vi "Test-DriveForwardDistance-DMR.vi"(9 "TestProgress NT":string, 10 "TestProgressText NT":string, 11 "TestName NT":string) -> ()   [LabVIEW 2013]
uses:
  Systems/DriveMotors/DriveMotors.lvclass
  Commands/DM-DriveForwardDistance/DM-DriveForwardDistance.lvclass
  Commands/Command/Command.lvclass
  Robot Global Data.vi
panel:
  in  "Test Wait":u32=25
  in  "DrivePower":dbl=0.4 format="%#_13g"
  in  "DistanceToDrive":dbl=600.0 format="%#_13g"
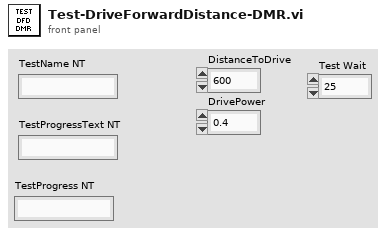
[diagram p1: front panel]
types:
  T1 = typedef "Semaphore RefNum" = refnum<k1>
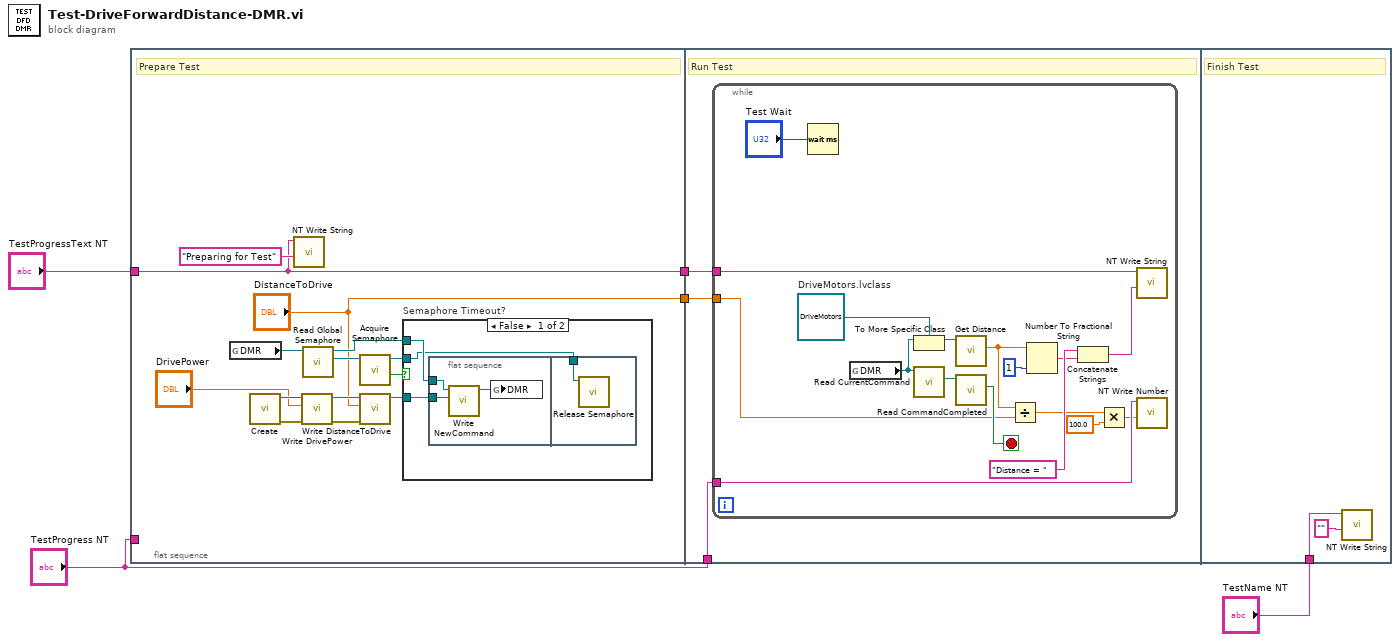
[diagram p0: block diagram]
diagram:
  n1 = flat-sequence {
    tunnel: "TestProgressText NT" -> [w8]
    tunnel: "TestProgress NT" -> [_]
    tunnel: [w8] -> w4
    tunnel: ["DistanceToDrive"] -> w3
    tunnel: w4 -> [w29]
    tunnel: w3 -> [w28]
    tunnel: "TestProgress NT" -> [w27]
    tunnel: "TestName NT" -> [w48]
    frame #0 {
      # "Prepare Test"
      n2 = global read "Robot Global Data.vi" "DMR"() -> (w16:refnum<class "DriveMotors.lvclass">)
      n3 = call "Create.vi"() -> ("error out"=w11:errorcluster, "DM-DriveForwardDistance.lvclass"=w19:refnum<class "DM-DriveForwardDistance.lvclass">)  [unwired: 10 in]
      n4 = call <vilib>:"NT Write String.vi"("String"="Preparing for Test", "Name"=w8) -> ()  [unwired: 9 in, 1 out]
      n5 = call-dynamic "Write DrivePower.vi"("error in (no error)"=w11, "DrivePower"="DrivePower", "DM-DriveForwardDistance in"=w19) -> ("error out"=w10:errorcluster, "DM-DriveForwardDistance out"=w18:refnum<class "DM-DriveForwardDistance.lvclass">)  [unwired: 7 in]
      n6 = call-dynamic "Read Global Semaphore.vi"("System in"=w16) -> ("semaphore"=w15:T1, "System out"=w13:refnum<class "DriveMotors.lvclass">)  [unwired: 8 in, 1 out]
      n7 = call <vilib>:"Acquire Semaphore.vi"("semaphore"=w15) -> ("timed out"=w14:bool, "semaphore out"=w12:T1)  [unwired: 4 in, 1 out]
      n8 = call-dynamic "Write DistanceToDrive.vi"("error in (no error)"=w10, "DistanceToDrive"="DistanceToDrive", "DM-DriveForwardDistance in"=w18) -> ("DM-DriveForwardDistance out"=w6:refnum<class "DM-DriveForwardDistance.lvclass">)  [unwired: 7 in, 1 out]
      n9 = case "Semaphore Timeout?" shown="False" w14 {
        tunnel: w13 -> [w22 _]
        tunnel: w6 -> [w21 _]
        tunnel: w12 -> [w20 _]
        frame False {
          n10 = flat-sequence {
            tunnel: w22 -> [w25]
            tunnel: w21 -> [w24]
            tunnel: w20 -> [w26]
            frame #0 {
              n11 = call-dynamic "Write NewCommand.vi"("Command.lvclass"=w24, "System in"=w25) -> ("System out"=w23:refnum<class "DriveMotors.lvclass">)  [unwired: 8 in, 1 out]
              n12 = global write "Robot Global Data.vi" "DMR"(w23) -> ()
            }
            frame #1 {
              n13 = call <vilib>:"Release Semaphore.vi"("semaphore"=w26) -> ()  [unwired: 5 in, 2 out]
            }
          }
        }
        frame True {
        }
      }
    }
    frame #1 {
      # "Run Test"
      n14 = while {
        tunnel: w29 -> [w45]
        tunnel: w28 -> [w37]
        tunnel: w27 -> [w35]
        stop <- w41 stop-if-true
        w39 = refnum<class "DriveMotors.lvclass"> refnum  # DriveMotors.lvclass
        n15 = Wait (ms)(milliseconds to wait="Test Wait") -> ()  [unwired: 1 out]
        n16 = global read "Robot Global Data.vi" "DMR"() -> (w40:refnum<class "DriveMotors.lvclass">)
        n17 = To More Specific Class(target class=w39, reference=w40) -> (specific class reference=w38:refnum<class "DriveMotors.lvclass">)  [unwired: 1 in, 1 out]
        n18 = call-dynamic "Read CurrentCommand.vi"("System in"=w40) -> ("Command.lvclass"=w42:refnum<class "Command.lvclass">)  [unwired: 8 in, 2 out]
        n19 = call-dynamic "Get Distance.vi"("DriveMotors in"=w38) -> ("Distance"=w34:dbl)  [unwired: 8 in, 2 out]
        n20 = call-dynamic "Read CommandCompleted.vi"("Command in"=w42) -> ("CommandCompleted"=w41:bool)  [unwired: 8 in, 2 out]
        n21 = Divide(x=w34, y=w37) -> (x/y=w36:dbl)
        n22 = Number To Fractional String(number=w34, precision (6)=i16 1) -> (F-format string=w33:string)  [unwired: 2 in]
        n23 = Concatenate Strings("Distance = " ("string"), w33) -> (w43:string)
        n24 = Multiply(x=w36, y=100.0) -> (x*y=w31:dbl)
        n25 = call <vilib>:"NT Write String.vi"("String"=w43, "Name"=w45) -> ()  [unwired: 9 in, 1 out]
        n26 = call <vilib>:"NT Write Number.vi"("Numeric"=w31, "Name"=w35) -> ()  [unwired: 9 in, 1 out]
      }
    }
    frame #2 {
      # "Finish Test"
      n27 = call <vilib>:"NT Write String.vi"("String"="", "Name"=w48) -> ()  [unwired: 9 in, 1 out]
    }
  }
